vi "Dashboard Main.vi"() -> ()   [LabVIEW 2016]
uses:
  <vilib>/Rock Robotics/Network Tables/NT Read Numeric Array.vi
  <vilib>/Rock Robotics/Network Tables/NT Read Number.vi
  <vilib>/Rock Robotics/Network Tables/NT Read Boolean.vi
panel:
  out "Camera Info":cluster{"Mbps LED":bool, "Mbps":dbl, "fps":dbl} {"fps" format="%#.1g"; "Mbps" format="%#.1g"}
  in  "Camera Settings":T1={"Frame Rate"=30, "Compression"=30, "Size"=1, "DB Camera Config"=FALSE} {"Frame Rate" scale=1.0..30.0; "Compression" scale=100.0..-1.0; "Size" items=["640x480", "320x240", "160x120"]}
  in  "TCP":refnum<k5>
  out "Robot IP":string
  in  "Dashboard Tab":enum32{"Drive", "Basic", "Custom", "Variables"}(tab)
  out "Controller 2":bool
  out "Controller 1":bool
  out "Reverse?":bool
  out "Ball Movers":bool
  out "Ball Direction":bool
  out "Drive Mode":bool
  out "Ultrasonic":u8(slide) caption="Slide" scale=0.0..40.0
  out "Enc Right":dbl
  out "Enc Left":dbl
  out "Gyro":dbl(knob) scale=0.0..360.0
  in  "Select Auto":string(combo)="Select Autonomous ..."
  out "NT Connection":bool
  out "MotorChart R":cluster{"Numeric":dbl, "Numeric":dbl}(graph)
  out "MotorChart L":cluster{"Numeric":dbl, "Numeric":dbl}(graph)
  out "MotorSliders R":cluster{"MotorSlide1":dbl, "MotorSlide2":dbl} {"MotorSlide2" scale=-1.0..1.0 scale format="%#_2e"; "MotorSlide1" scale=-1.0..1.0 scale format="%#_2e"}
  out "MotorSliders L":cluster{"MotorSlide1":dbl, "MotorSlide2":dbl} {"MotorSlide2" scale=-1.0..1.0 scale format="%#_2e"; "MotorSlide1" scale=-1.0..1.0 scale format="%#_2e"}
  out "JS1 Z":dbl(slide) scale=-1.0..1.0 scale format="%#_2e"
  out "JS1 Graph":cluster{"X":dbl, "Y":dbl}[](graph)
  out "JS1 Buttons":T2
  out "JS2 Z":dbl(slide) scale=-1.0..1.0 scale format="%#_2e"
  out "JS2 Graph":cluster{"X":dbl, "Y":dbl}[](graph)
  out "JS2 Buttons":T2
  out "Mode":T3(ring)=enum."Auto Disabled"
  in  "DB/String 9":string
  in  "DB/String 8":string
  in  "DB/String 7":string
  in  "DB/String 6":string
  in  "DB/String 5":string
  in  "DB/String 4":string
  in  "DB/String 3":string
  in  "DB/String 2":string
  in  "DB/String 1":string
  in  "DB/String 0":string
  in  "DB/Slider 0":dbl(slide) scale=0.0..5.0
  in  "DB/Slider 1":dbl(slide) scale=0.0..5.0
  in  "DB/Slider 2":dbl(slide) scale=0.0..5.0
  in  "DB/Slider 3":dbl(slide) scale=0.0..5.0
  out "DB/LED 3":bool
  out "DB/LED 2":bool
  out "DB/LED 1":bool
  out "DB/LED 0":bool
  in  "DB/Button 3":bool
  in  "DB/Button 2":bool
  in  "DB/Button 1":bool
  in  "DB/Button 0":bool caption="New Name"
  out "Tree":string(tree)
  out "Camera Image":T4(plugin-control)
  out "Background":bool
  in  "Camera Name":string(combo)="No Camera Selection"
  # "HW"
  # "Joysticks"
  # "Drive Motors"
  # "Front"
  # "Right"
  # "Left"
  # "Back"
  # "This tab is a great place for autonomous settings and robot-specific values.\nPlace controls and indicators inside this tab and match name to\nDashboard Variables on robot. You can also delete this comment."
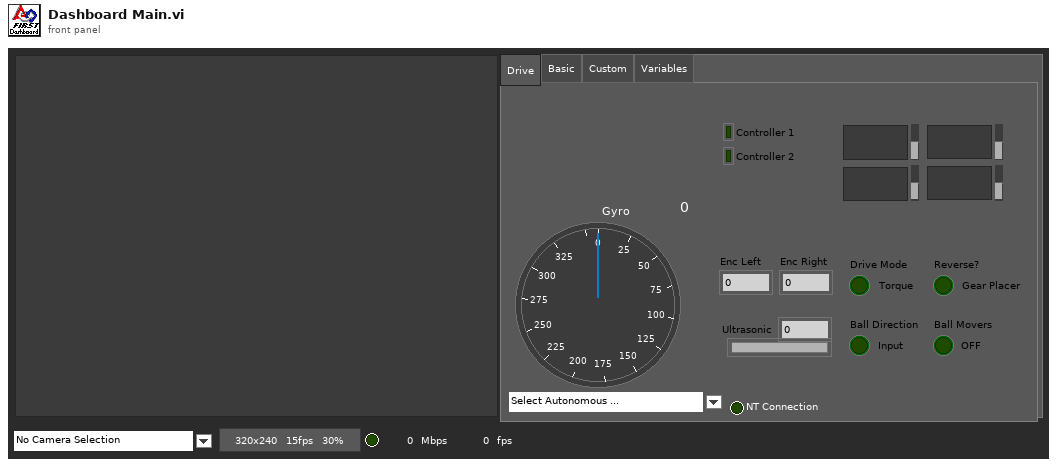
[diagram p1: front panel]
types:
  T1 = cluster{"Frame Rate":i32, "Compression":i32, "Size":u16, "DB Camera Config":bool}
  T2 = cluster{bool, bool, bool, bool, bool, bool, bool, bool, bool, bool, bool, bool}
  T3 = enum8{"Tele-Op Disabled", "Tele-Op Enabled", "Auto Disabled", "Auto Enabled", "Test Disabled", "Test Enabled", "Disconnected", "No Code", "E-Stop"}
  T4 = typedef "IMAQ Image.ctl" = refnum<image>
  T5 = enum32{"Drive", "Basic", "Custom", "Test", "Checklist", "Variables"}
  T6 = typedef "Image Type" = u32
  T7 = cluster{"Camera Image":refnum<vi>, "Dashboard Tab":refnum<vi>, "Background":refnum<vi>, "Tree":refnum<vi>, "Camera Settings":refnum<vi>, "Camera Name":refnum<vi>, "Camera Info":refnum<vi>}
  T8 = cluster{"Shift":bool, "Ctrl":bool, "Alt":bool, "Cmd":bool, "Opt":bool}
  T9 = cluster{"Error Strings":string, "Disable Counts":cluster{u16, u16}, "Rail Faults":cluster{u16, u16, u16}, "Robot IP":string, "DB Mode":u8, "Event Info":cluster{"Name":string, "Type":u8, "Number":u16, "Replay":u8}}
  T10 = cluster{"Storage":cluster{"Disk Free":u64, "RAM Block":u32, "RAM free":u32}, "CPU Utilization":cluster{"CPU % ISR":sgl, "CPU % Time Crit":sgl, "CPU % Timed Str":sgl, "CPU % High":sgl, "CPU % Above":sgl, "CPU % Normal":sgl, "CPU % Low":sgl}, "CAN":cluster{"% Bus Utilization":sgl, "Bus Off Cnt":u32, "TX_FIFO Full Cnt":u32, "Receive Error Cnt":u8, "Transmit Error Cnt":u8}, "HID":cluster{"HID Outputs":u32, "Rumble Low":u16, "Rumble High":u16}[]}
  T11 = cluster{"Status bits":cluster{"Test Mode":bool, "Autonomous":bool, "Enabled":bool, "Code Start":bool, "Brownout":bool, "Reserved 2":bool, "Reserved 3":bool, "E-Stop":bool}, "Code Trace":cluster{"Disabled":bool, "TeleOp":bool, "Auto":bool, "Test":bool}, "Controller Type":enum16{"unknown", "cRIO", "roboRio"}, "Code?":enum16{"unknown", "noCode", "code"}, "Battery V":dbl}
  T12 = cluster{"Control Bits":cluster{"TestMode":bool, "Autonomous":bool, "Enabled":bool, "FMS Present":bool, bool, bool, bool, "E-Stop":bool}, "Team Station ":u8, "Countdown":sgl, "Joystick Values":cluster{"Axes":dbl[], "Buttons":bool[], "POVs":i16[]}[]}
  T13 = cluster{"Axes":dbl[], "Buttons":bool[], "POVs":i16[]}[]
  T14 = cluster{"Axes":dbl[], "Buttons":bool[], "POVs":i16[]}
  T15 = cluster{"Buttons[0]":bool, "Buttons[1]":bool, "Buttons[2]":bool, "Buttons[3]":bool, "Buttons[4]":bool, "Buttons[5]":bool, "Buttons[6]":bool, "Buttons[7]":bool, "Buttons[8]":bool, "Buttons[9]":bool, "Buttons[10]":bool, "Buttons[11]":bool}
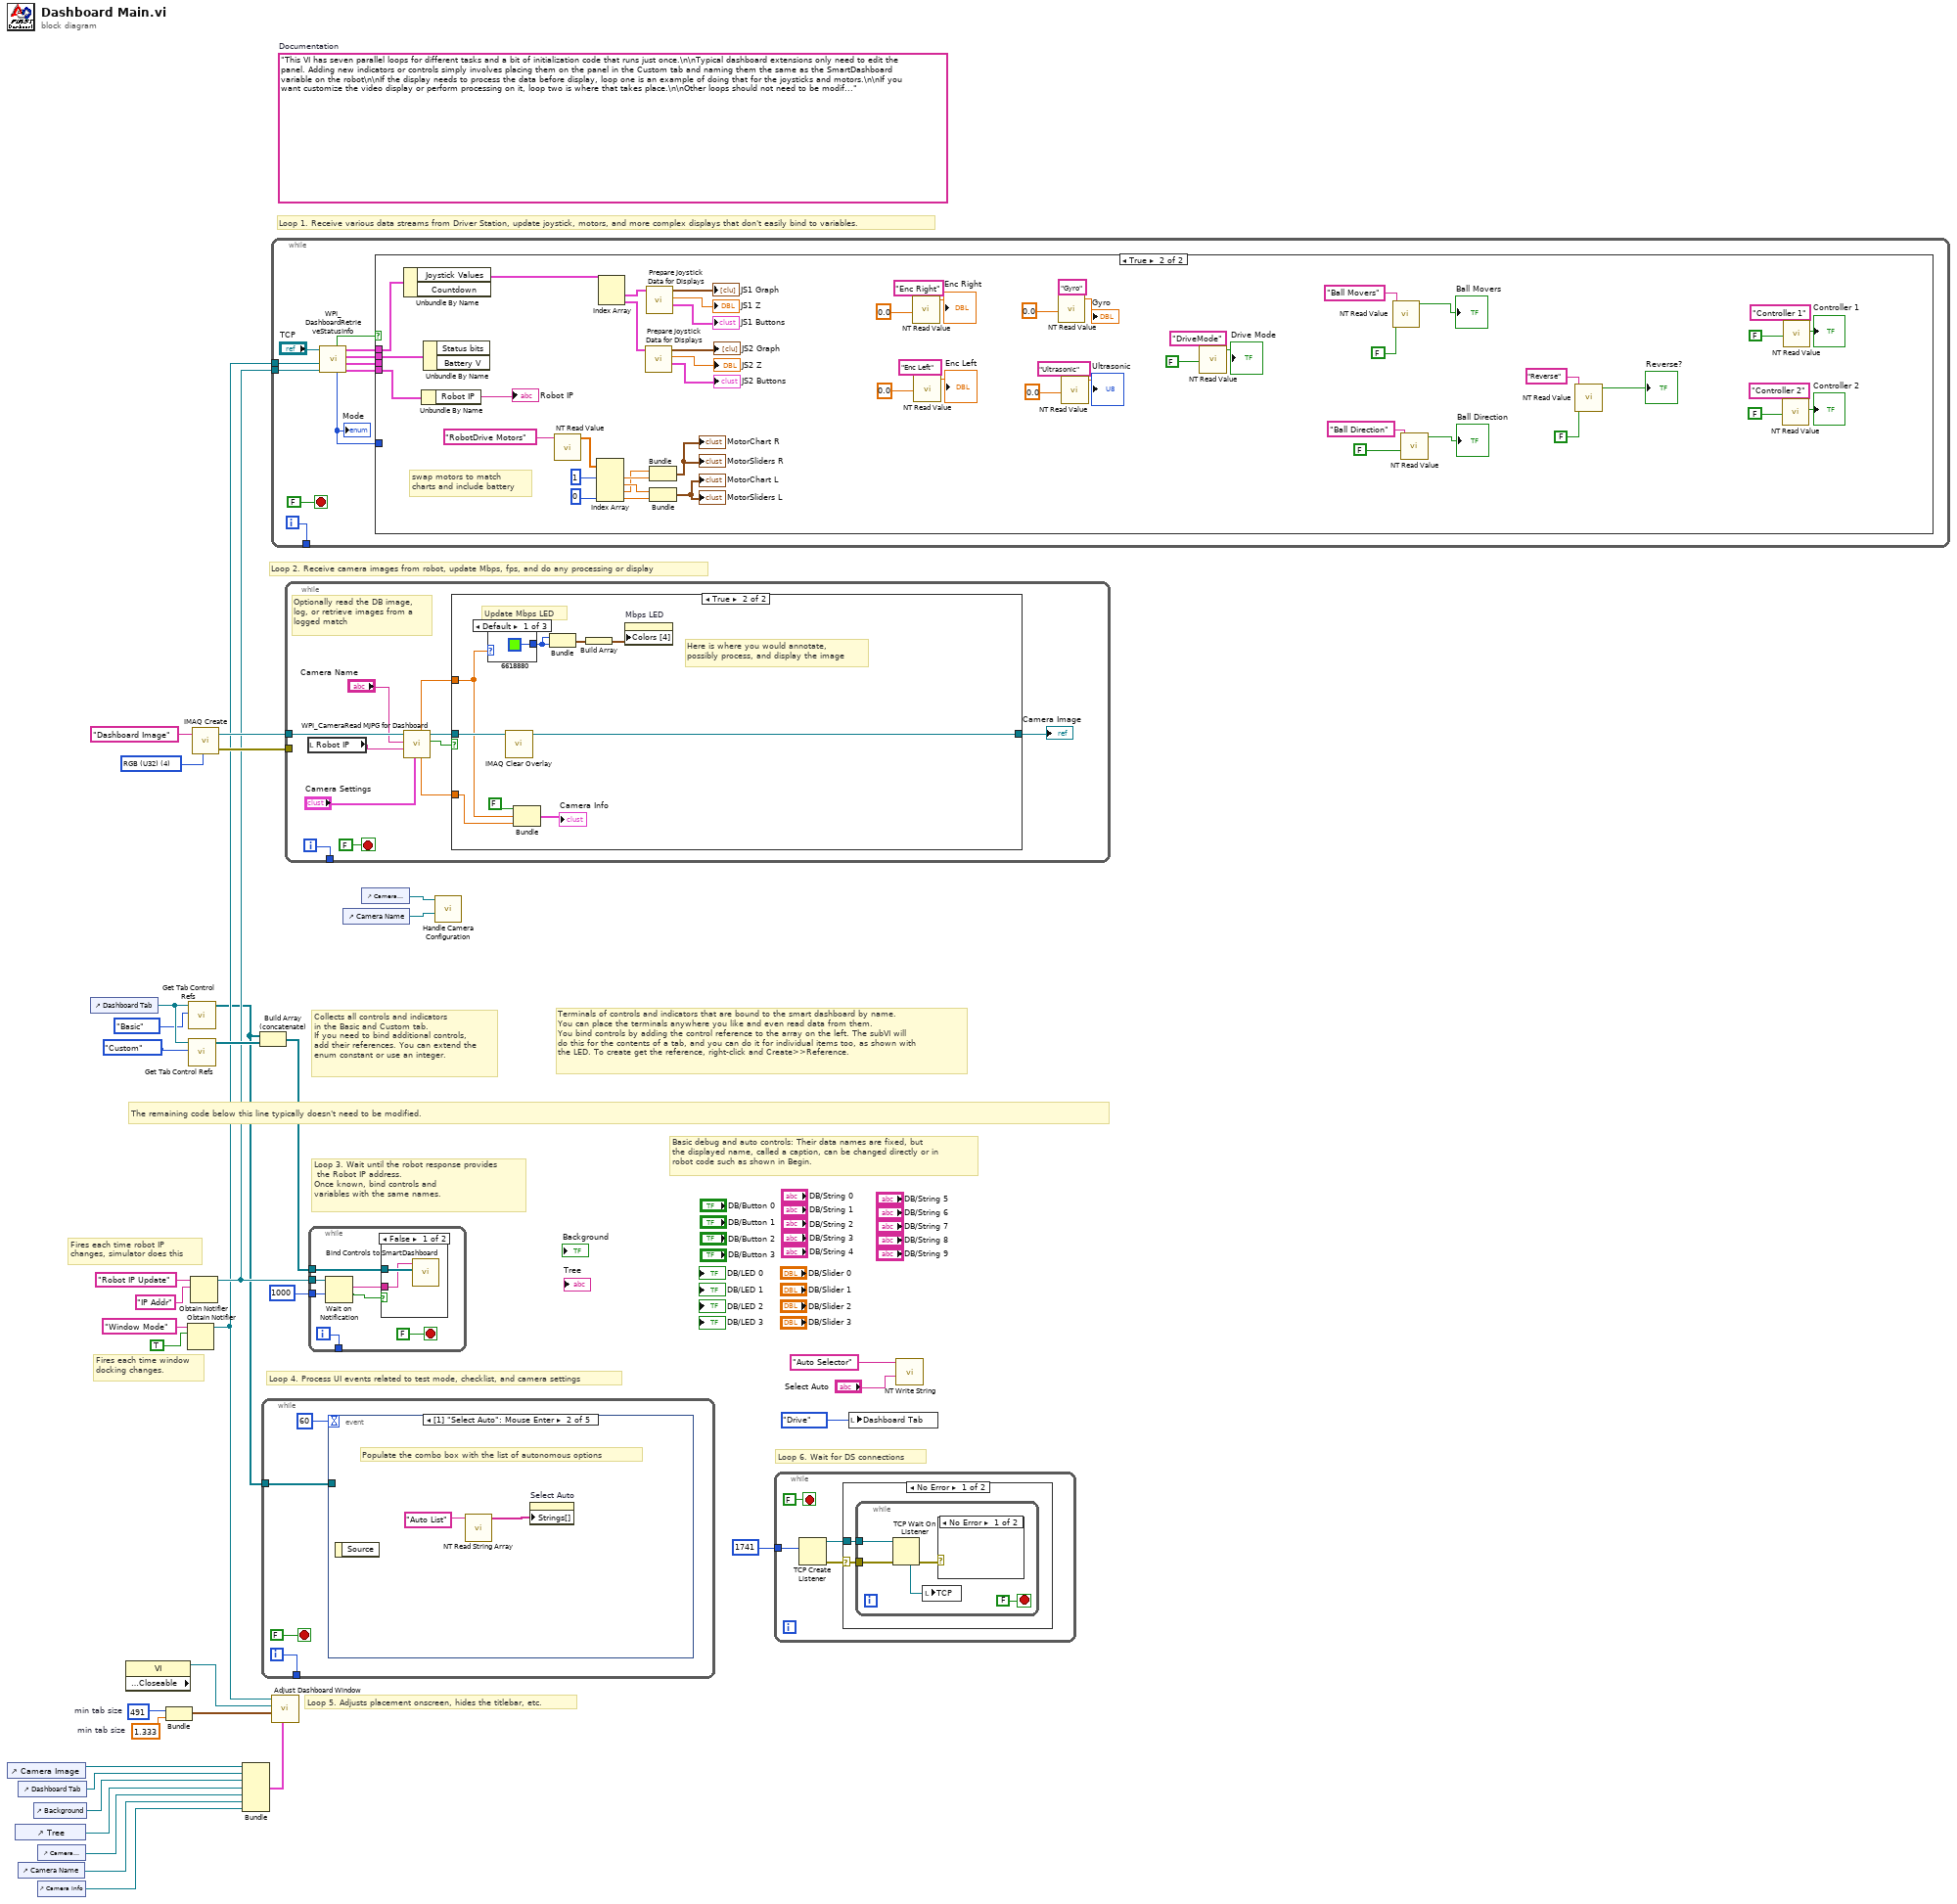
[diagram p0: block diagram]
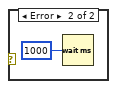
[diagram p2: hidden frame]
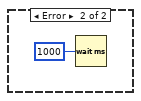
[diagram p3: hidden frame]
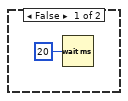
[diagram p4: hidden frame]
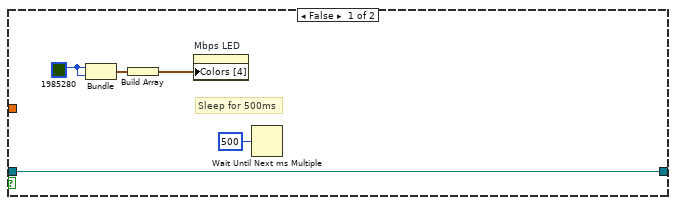
[diagram p6: hidden frame]
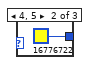
[diagram p7: hidden frame]
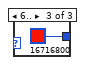
[diagram p8: hidden frame]
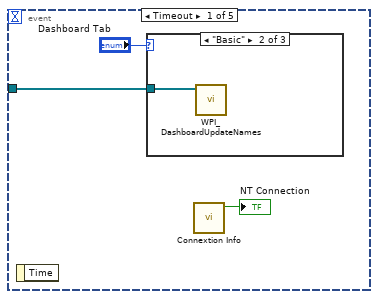
[diagram p9: hidden frame]
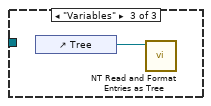
[diagram p11: hidden frame]
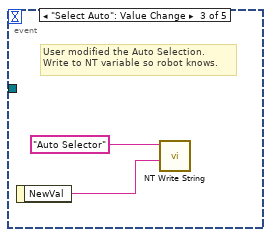
[diagram p12: hidden frame]
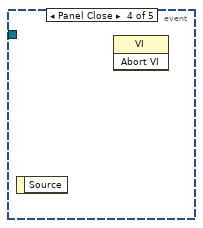
[diagram p13: hidden frame]
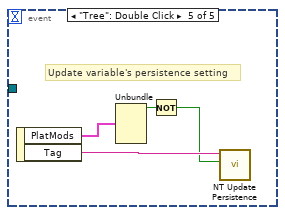
[diagram p14: hidden frame]
diagram:
  w20 = 491  # min tab size
  w19 = 1.333  # min tab size
  (unwired) "This VI has seven parallel loops for different tasks and a bit of initialization code that runs just once.\n\nTypical dashboard extensions only need to edit the panel. Adding new indicators or controls simply involves placing them on the panel in the Custom tab and naming them the same as the SmartDashboard variable on the robot\n\nIf the display needs to process the data before display, loop one is an example of doing that for the joysticks and motors.\n\nIf you want customize the video display or perform processing on it, loop two is where that takes place.\n\nOther loops should not need to be modified. They are pretty standard, and document the task they perform."  # Documentation
  w35 = T6 4 items=["Grayscale (U8)", "Grayscale (I16)", "Grayscale (SGL)", "Complex (CSG)", "RGB (U32)", "HSL (U32)", "RGB (U64)"] ("Image Type")
  # "Loop 6. Wait for DS connections"
  # "Basic debug and auto controls: Their data names are fixed, but\nthe displayed name, called a caption, can be changed directly or in\nrobot code such as shown in Begin."
  # "Fires each time robot IP\nchanges, simulator does this"
  # "Fires each time window\ndocking changes."
  # "Collects all controls and indicators\nin the Basic and Custom tab.\nIf you need to bind additional controls,\nadd their references. You can extend the\nenum constant or use an integer."
  # "The remaining code below this line typically doesn't need to be modified."
  # "Loop 4. Process UI events related to test mode, checklist, and camera settings"
  # "Terminals of controls and indicators that are bound to the smart dashboard by name.\nYou can place the terminals anywhere you like and even read data from them.\nYou bind controls by adding the control reference to the array on the left. The subVI will\ndo this for the contents of a tab, and you can do it for individual items too, as shown with\nthe LED. To create get the reference, right-click and Create>>Reference."
  # "Loop 3. Wait until the robot response provides\n the Robot IP address.\nOnce known, bind controls and\nvariables with the same names."
  # "Loop 5. Adjusts placement onscreen, hides the titlebar, etc."
  # "Loop 1. Receive various data streams from Driver Station, update joystick, motors, and more complex displays that don't easily bind to variables."
  # "Loop 2. Receive camera images from robot, update Mbps, fps, and do any processing or display"
  n1 = control-ref of="Camera Image"() -> (w22:refnum<vi>)
  n2 = control-ref of="Tree"() -> (w4:refnum<vi>)
  n3 = control-ref of="Dashboard Tab"() -> (w21:refnum<vi>)
  n4 = control-ref of="Camera Name"() -> (w2:refnum<vi>)
  n5 = control-ref of="Background"() -> (w17:refnum<vi>)
  n6 = control-ref of="Camera Settings"() -> (w3:refnum<vi>)
  n7 = control-ref of="Camera Info"() -> (w1:refnum<vi>)
  n8 = control-ref of="Dashboard Tab"() -> (w25:refnum<vi>)
  n9 = property class="VI" props=["Front Panel.Closeable"]() -> (reference out=w26:refnum<vi>)  [unwired: 2 in, 2 out]
  n10 = Bundle("min tab size"=w20, "min tab size"=w19) -> (w18:cluster{"min tab size":i32, "min tab size":dbl})  [unwired: 1 in]
  n11 = Obtain Notifier(name (unnamed)="Window Mode", notification data type=TRUE) -> (notifier out=w12:refnum<notifier>)  [unwired: 2 in, 2 out]
  n12 = call <vilib>:"Get Tab Control Refs.vi"("Page Index"=T5."Basic" ("Dashboard Tab"), "TabControl in"=w25) -> ("ControlsOnPage"=w7:refnum<vi>[])  [unwired: 9 in]
  n13 = call <vilib>:"Get Tab Control Refs.vi"("Page Index"=T5."Custom" ("Dashboard Tab"), "TabControl in"=w25) -> ("ControlsOnPage"=w24:refnum<vi>[])  [unwired: 9 in]
  n14 = Obtain Notifier(name (unnamed)="Robot IP Update", notification data type="IP Addr" ("name (unnamed)")) -> (notifier out=w13:refnum<notifier>)  [unwired: 2 in, 2 out]
  n15 = call "IMAQ Create"("Image Name"="Dashboard Image", "Image Type"=w35) -> ("New Image"=w33:T4, "error out"=w32:errorcluster)  [unwired: 2 in, 1 out]
  n16 = Bundle("Camera Image"=w22, "Dashboard Tab"=w21, "Background"=w17, "Tree"=w4, "Camera Settings"=w3, "Camera Name"=w2, "Camera Info"=w1) -> (w14:T7)  [unwired: 1 in]
  n17 = Build Array (concatenate)(w7, w24) -> (w23:refnum<vi>[])
  n18 = while {
    tunnel: [w37] -> _
    tunnel: w7 -> [w36]
    i -> [w37]
    stop <- FALSE stop-if-true
    n19 = event shown="[1] \"Select Auto\": Mouse Enter" {
      selector: _ -> [_ _ _ _ _]
      dyn-events: _ -> [_ _ _ _ _]
      timeout: u32 60 ("milliseconds to wait") -> [_ _ _ _ _]
      tunnel: w36 -> [w40 _ _ _ _]
      event Timeout {
        n20 = event-data() -> ()  [unwired: 1 in, 1 out]
        n21 = case shown="\"Basic\"" "Dashboard Tab" {
          tunnel: w40 -> [_ w43 _]
          frame "Custom", Default {
          }
          frame "Basic" {
            n22 = call <vilib>:"WPI_DashboardUpdateNames.vi"("Controls on Tab"=w43) -> ()  [unwired: 11 in]
          }
          frame "Variables" {
            n23 = control-ref of="Tree"() -> (w44:refnum<vi>)
            n24 = call <vilib>:"NT Read and Format Entries as Tree.vi"("Tree Refnum"=w44) -> ()  [unwired: 9 in, 2 out]
          }
        }
        n25 = call <vilib>:"Connextion Info.vi"() -> ("Connected"=→"NT Connection":bool)  [unwired: 10 in, 1 out]
      }
      event "Select Auto": Mouse Enter {
        # "Populate the combo box with the list of autonomous options"
        n26 = event-data() -> ()  [unwired: 1 in, 1 out]
        n27 = call <vilib>:"NT Read String Array.vi"("Name"="Auto List") -> ("String Array"=w45:string[])  [unwired: 9 in, 1 out]
        n28 = property on="Select Auto" class="CmbBox"("Strings[]"=w45) -> ()  [unwired: 2 in, 2 out]
      }
      event "Select Auto": Value Change {
        # "User modified the Auto Selection.\nWrite to NT variable so robot knows."
        n29 = event-data() -> ("NewVal"=w47:string)  [unwired: 1 in]
        n30 = call <vilib>:"NT Write String.vi"("String"=w47, "Name"="Auto Selector") -> ()  [unwired: 9 in, 1 out]
      }
      event Panel Close {
        n31 = event-data() -> ()  [unwired: 1 in, 1 out]
        n32 = invoke class="VI" method="Abort VI"() -> ()  [unwired: 3 in, 3 out]
      }
      event "Tree": Double Click {
        # "Update variable's persistence setting"
        n33 = event-data() -> ("PlatMods"=w52:T8, "Tag"=w51:string)  [unwired: 1 in]
        n34 = Unbundle(w52) -> ("Shift"=w50:bool)  [unwired: 4 out]
        n35 = Not(x=w50) -> (.not. x?=w49:bool)
        n36 = call <vilib>:"NT Update Persistence.vi"("Persistence"=w49, "Name"=w51) -> ()  [unwired: 9 in, 1 out]
      }
    }
  }
  n37 = while {
    tunnel: [w62] -> _
    tunnel: w13 -> [w56]
    tunnel: w12 -> [w53]
    i -> [w62]
    stop <- FALSE stop-if-true
    n38 = call <vilib>:"WPI_DashboardRetrieveStatusInfo.vi"("Binding Refnum"=w56, "Window Mode Notifier"=w53, "TCP Cnx"="TCP") -> ("Power and Errors"=w57:T9, "Robot Metrics"=w60:T10, "Status Info"=w61:T11, "Control Info"=w58:T12, "Robot Mode"=w55:T3, "Process?"=w59:bool)  [unwired: 3 in]
    "Mode" <- w55
    n39 = case shown="True" w59 {
      tunnel: w61 -> [_ w117]
      tunnel: w60 -> [_ _]
      tunnel: w58 -> [_ w116]
      tunnel: w57 -> [_ w115]
      tunnel: w55 -> [_ _]
      frame False {
        n40 = Wait (ms)(milliseconds to wait=u32 20) -> ()  [unwired: 1 out]
      }
      frame True {
        # "swap motors to match\ncharts and include battery"
        n41 = Unbundle By Name(w116) -> ("Joystick Values"=w106:T13)  [unwired: 1 out]
        n42 = Unbundle By Name(w115) -> ("Robot IP"=→"Robot IP":string)
        n43 = Unbundle By Name(w117) -> ()  [unwired: 2 out]
        n44 = call-poly <vilib>:"NT Read Value.vi"("Name"="RobotDrive Motors") -> ("Numeric Array"=w96:dbl[])  [unwired: 9 in, 1 out]
        n45 = Index Array(array=w96, index #1=1, index #4=0) -> (element #1=w110:dbl, element #2=w111:dbl, element #3=w109:dbl, element #4=w114:dbl)  [unwired: 2 in]
        n46 = Index Array(array=w106) -> (element #1=w105:T14, element #2=w101:T14)  [unwired: 2 in]
        n47 = call "Prepare Joystick Data for Displays.vi"("Joystick Values"=w101) -> ("Buttons"=→"JS2 Buttons":T15, "Z Axis"=→"JS2 Z":dbl, "Cartesian Data"=→"JS2 Graph":cluster{"X axis":dbl, "X axis":dbl}[])  [unwired: 8 in]
        n48 = call "Prepare Joystick Data for Displays.vi"("Joystick Values"=w105) -> ("Buttons"=→"JS1 Buttons":T15, "Z Axis"=→"JS1 Z":dbl, "Cartesian Data"=→"JS1 Graph":cluster{"X axis":dbl, "X axis":dbl}[])  [unwired: 8 in]
        n49 = Bundle("Numeric"=w109, "Numeric"=w110) -> (→"MotorChart R" →"MotorSliders R":cluster{"Numeric":dbl, "Numeric":dbl})  [unwired: 1 in]
        n50 = Bundle("Numeric"=w111, "Numeric"=w114) -> (→"MotorChart L" →"MotorSliders L":cluster{"Numeric":dbl, "Numeric":dbl})  [unwired: 1 in]
        n51 = call-poly <vilib>:"NT Read Value.vi"("Default Value"=0.0, "Name"="Enc Right") -> ("Numeric"=→"Enc Right":dbl)  [unwired: 8 in, 1 out]
        n52 = call-poly <vilib>:"NT Read Value.vi"("Default Value"=0.0, "Name"="Enc Left") -> ("Numeric"=→"Enc Left":dbl)  [unwired: 8 in, 1 out]
        n53 = call-poly <vilib>:"NT Read Value.vi"("Default Value"=0.0, "Name"="Gyro") -> ("Numeric"=→"Gyro":dbl)  [unwired: 8 in, 1 out]
        n54 = call-poly <vilib>:"NT Read Value.vi"("Default Value"=0.0, "Name"="Ultrasonic") -> ("Numeric"=→"Ultrasonic":dbl)  [unwired: 8 in, 1 out]
        n55 = call-poly <vilib>:"NT Read Value.vi"("Default Value"=FALSE, "Name"="DriveMode") -> ("Boolean"=→"Drive Mode":bool)  [unwired: 8 in, 1 out]
        n56 = call-poly <vilib>:"NT Read Value.vi"("Default Value"=FALSE, "Name"="Ball Movers") -> ("Boolean"=→"Ball Movers":bool)  [unwired: 8 in, 1 out]
        n57 = call-poly <vilib>:"NT Read Value.vi"("Default Value"=FALSE, "Name"="Ball Direction") -> ("Boolean"=→"Ball Direction":bool)  [unwired: 8 in, 1 out]
        n58 = call-poly <vilib>:"NT Read Value.vi"("Default Value"=FALSE, "Name"="Reverse") -> ("Boolean"=→"Reverse?":bool)  [unwired: 8 in, 1 out]
        n59 = call-poly <vilib>:"NT Read Value.vi"("Default Value"=FALSE, "Name"="Controller 2") -> ("Boolean"=→"Controller 2":bool)  [unwired: 8 in, 1 out]
        n60 = call-poly <vilib>:"NT Read Value.vi"("Default Value"=FALSE, "Name"="Controller 1") -> ("Boolean"=→"Controller 1":bool)  [unwired: 8 in, 1 out]
      }
    }
  }
  n61 = call "Adjust Dashboard Window.vi"("Sizing Refnums"=w14, "Size Constraints"=w18, "VI"=w26, "WIn Mode"=w12) -> ()  [unwired: 8 in]
  n62 = while {
    tunnel: w33 -> [w126]
    tunnel: w32 -> [_]
    tunnel: [w127] -> _
    i -> [w127]
    stop <- FALSE stop-if-true
    # "Optionally read the DB image,\nlog, or retrieve images from a\nlogged match"
    n63 = local read "Robot IP"() -> (w122:string)
    n64 = call <vilib>:"WPI_CameraRead MJPG for Dashboard.vi"("Camera Settings"="Camera Settings", "Robot IP"=w122, "Camera Name"="Camera Name", "Refnum in"=w126) -> ("Active"=w124:bool, "Refnum out"=w125:T4, "FPS"=w123:dbl, "Bandwidth (Mbps)"=w121:dbl)  [unwired: 4 in]
    n65 = case shown="True" w124 {
      tunnel: w125 -> [w129 w140]
      tunnel: w121 -> [_ w137]
      tunnel: w123 -> [_ w138]
      tunnel: [w129 w134] -> w118
      frame False {
        w131 = u32 1985280 ("Color Box")
        # "Sleep for 500ms"
        n66 = Bundle("Color Box"=w131, "Color Box"=w131) -> (w132:cluster{"Color Box":u32, "Color Box":u32})  [unwired: 1 out]
        n67 = Build Array(w132) -> (w130:cluster{"Color Box":u32, "Color Box":u32}[])
        n68 = property on="Mbps LED" class="Bool (strict)"("Colors [4]"=w130) -> ()  [unwired: 2 in, 2 out]
        n69 = Wait Until Next ms Multiple(millisecond multiple=u32 500) -> ()  [unwired: 1 out]
      }
      frame True {
        # "Here is where you would annotate,\npossibly process, and display the image"
        # "Update Mbps LED"
        n70 = case shown="Default" w137 {
          tunnel: [u32 6618880 ("Color Box") u32 16776722 ("Color Box") u32 16716800 ("Color Box")] -> w141
          frame Default {
          }
          frame 4, 5 {
          }
          frame 6.. {
          }
        }
        n71 = call "IMAQ Clear Overlay"("Image"=w140) -> ("Image Out"=w134:T4)  [unwired: 2 in, 8 out]
        n72 = Bundle(FALSE, "Bandwidth (Mbps)"=w137, "FPS"=w138) -> (→"Camera Info":cluster{bool, "Bandwidth (Mbps)":dbl, "FPS":dbl})  [unwired: 1 in]
        n73 = Bundle("Color Box"=w141, "Color Box"=w141) -> (w142:cluster{"Color Box":u32, "Color Box":u32})  [unwired: 1 out]
        n74 = Build Array(w142) -> (w139:cluster{"Color Box":u32, "Color Box":u32}[])
        n75 = property on="Mbps LED" class="Bool (strict)"("Colors [4]"=w139) -> ()  [unwired: 2 in, 2 out]
      }
    }
    "Camera Image" <- w118
  }
  n76 = while {
    tunnel: w23 -> [w152]
    tunnel: w13 -> [w150]
    tunnel: [w148] -> _
    tunnel: u32 1000 ("milliseconds to wait") -> [w147]
    i -> [w148]
    stop <- FALSE stop-if-true
    n77 = Wait on Notification(notifier=w150, timeout in ms (-1)=w147) -> (notification=w149:string, timed out?=w146:bool)  [unwired: 2 in, 2 out]
    n78 = case shown="False" w146 {
      tunnel: w152 -> [w154 _]
      tunnel: w149 -> [w153 _]
      frame False {
        n79 = call <vilib>:"Bind Controls to SmartDashboard.vi"("Bound Control Refs"=w154, "Server IP Address"=w153) -> ()  [unwired: 10 in]
      }
      frame True {
      }
    }
  }
  n80 = control-ref of="Camera Name"() -> (w8:refnum<vi>)
  n81 = control-ref of="Camera Settings"() -> (w9:refnum<vi>)
  n82 = call "Handle Camera Configuration.vi"("CameraNameRef"=w8, "ClusterRef"=w9) -> ()  [unwired: 10 in]
  n83 = while {
    tunnel: u16 1741 ("timeout ms (25000)") -> [w156]
    stop <- FALSE stop-if-true
    n84 = TCP Create Listener(10:w156) -> (0:w155:errorcluster, 3:w157:refnum<k5>)  [unwired: 4 in, 1 out]
    n85 = case shown="No Error" w155 {
      selector: w155 -> [w159 _]
      tunnel: w157 -> [w160 _]
      frame No Error {
        n86 = while {
          tunnel: w160 -> [w163]
          tunnel: w159 -> [w162]
          stop <- FALSE stop-if-true
          n87 = TCP Wait On Listener(8:w162, 11:w163) -> (0:w164:errorcluster, 4:w165:refnum<k5>)  [unwired: 2 in, 3 out]
          n88 = local write "TCP"(w165) -> ()
          n89 = case shown="No Error" w164 {
            frame No Error {
            }
            frame Error {
              n90 = Wait (ms)(milliseconds to wait=u32 1000) -> ()  [unwired: 1 out]
            }
          }
        }
      }
      frame Error {
        n91 = Wait (ms)(milliseconds to wait=u32 1000) -> ()  [unwired: 1 out]
      }
    }
  }
  n92 = local write "Dashboard Tab"(enum32{"Drive", "Basic", "Custom", "Variables"}."Drive" ("Dashboard Tab")) -> ()
  n93 = call <vilib>:"NT Write String.vi"("String"="Select Auto", "Name"="Auto Selector") -> ()  [unwired: 9 in, 1 out]
